vi "Get occupied squares by color.vi"(10 "Color":T4, 11 "Board in":refnum<class "Board.lvclass">) -> (2 "Squares":T1[](array[typedef]), 3 "Board out":refnum<class "Board.lvclass">)   [LabVIEW 2015, in "Chesslib.lvlib" / "Board.lvclass"]
uses:
  Board.lvclass
  typedef/Color.ctl
  typedef/Square.ctl
  typedef/File.ctl
  typedef/Rank.ctl
  Board.lvclass/Board.ctl
  Pieces/Piece/Piece.lvclass
  Chesslib.lvlib
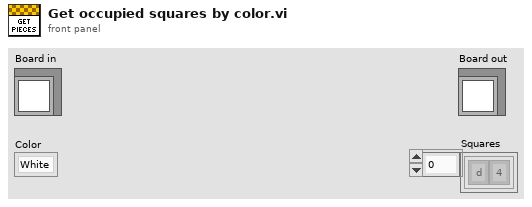
[diagram p1: front panel]
types:
  T1 = typedef "Chesslib.lvlib/Square.ctl" = cluster{"File":T2, "Rank":T3}
  T2 = typedef "Chesslib.lvlib/File.ctl" = enum16{"a", "b", "c", "d", "e", "f", "g", "h"}
  T3 = typedef "Chesslib.lvlib/Rank.ctl" = enum16{"1", "2", "3", "4", "5", "6", "7", "8"}
  T4 = typedef "Chesslib.lvlib/Color.ctl" = enum16{"White", "Black"}
  T5 = cluster{"Occupied":bool, "Piece":refnum<class "Piece.lvclass">}[]
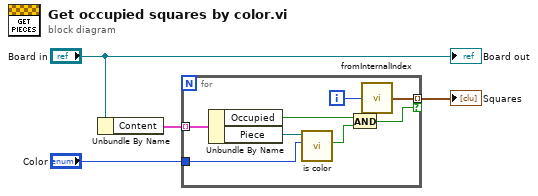
[diagram p0: block diagram]
diagram:
  n1 = Unbundle By Name("Board in") -> ("Content"=w3:T5)
  n2 = for {
    tunnel: w3 -> [w12] mode=indexing
    tunnel: "Color" -> [w10]
    tunnel: [w5] -> w1 mode=indexing if=w6
    i -> [w7]
    n3 = Unbundle By Name(w12) -> ("Occupied"=w8:bool, "Piece"=w11:refnum<class "Piece.lvclass">)
    n4 = call "is color.vi"("Color"=w10, "Piece in"=w11) -> ("is color?"=w9:bool)  [unwired: 9 in]
    n5 = And(x=w8, y=w9) -> (x .and. y?=w6:bool)
    n6 = call "fromInternalIndex.vi"("Internal index"=w7) -> ("Square"=w5:T1)
  }
  "Squares" <- w1
  "Board out" <- "Board in"
